vi "GetPDPCurrents.vi"() -> (2 "PDP Currents":dbl[](array[numeric]))   [LabVIEW 2016]
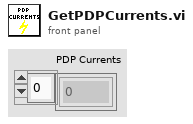
[diagram p1: front panel]
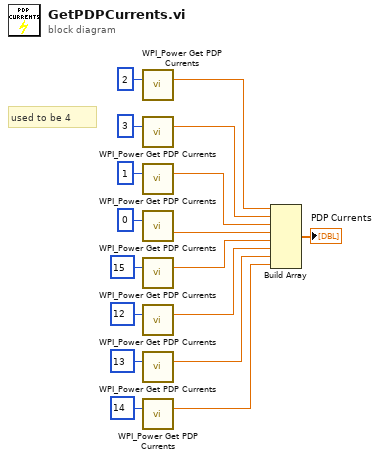
[diagram p0: block diagram]
diagram:
  # "used to be 4"
  n1 = call <vilib>:"WPI_Power Get PDP Currents.vi"("PDP Channel"=2) -> ("current (A)"=w9:dbl)  [unwired: 12 in, 2 out]
  n2 = call <vilib>:"WPI_Power Get PDP Currents.vi"("PDP Channel"=3) -> ("current (A)"=w8:dbl)  [unwired: 12 in, 2 out]
  n3 = call <vilib>:"WPI_Power Get PDP Currents.vi"("PDP Channel"=1) -> ("current (A)"=w7:dbl)  [unwired: 12 in, 2 out]
  n4 = call <vilib>:"WPI_Power Get PDP Currents.vi"("PDP Channel"=0) -> ("current (A)"=w6:dbl)  [unwired: 12 in, 2 out]
  n5 = call <vilib>:"WPI_Power Get PDP Currents.vi"("PDP Channel"=15) -> ("current (A)"=w5:dbl)  [unwired: 12 in, 2 out]
  n6 = call <vilib>:"WPI_Power Get PDP Currents.vi"("PDP Channel"=12) -> ("current (A)"=w4:dbl)  [unwired: 12 in, 2 out]
  n7 = call <vilib>:"WPI_Power Get PDP Currents.vi"("PDP Channel"=13) -> ("current (A)"=w3:dbl)  [unwired: 12 in, 2 out]
  n8 = call <vilib>:"WPI_Power Get PDP Currents.vi"("PDP Channel"=14) -> ("current (A)"=w2:dbl)  [unwired: 12 in, 2 out]
  n9 = Build Array(w9, w8, w7, w6, w5, w4, w3, w2) -> (→"PDP Currents":dbl[])
